vi "normalise_3d_vector.vi"(3 "Vector":cluster{dbl, dbl, dbl}) -> (0 "Unit Vector":cluster{dbl, dbl, dbl}, 1 "magnitude":dbl)   [LabVIEW 2019]
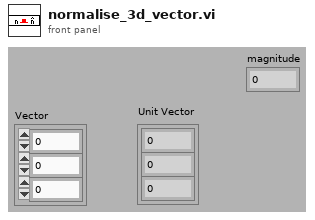
[diagram p1: front panel]
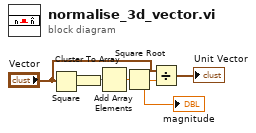
[diagram p0: block diagram]
diagram:
  n1 = Square(x="Vector") -> (x^2=w1:cluster{dbl, dbl, dbl})
  n2 = Cluster To Array(cluster=w1) -> (array=w2:dbl[])
  n3 = Add Array Elements(numeric array=w2) -> (sum=w3:dbl)
  n4 = Square Root(x=w3) -> (sqrt(x)=w4:dbl)
  "magnitude" <- w4
  n5 = Divide(x="Vector", y=w4) -> (x/y=→"Unit Vector":cluster{dbl, dbl, dbl})
